vi "Calculator.vi"() -> ()   [LabVIEW 2014]
panel:
  in  ".":bool
  in  "=":bool
  in  "0":bool
  in  "3":bool
  in  "2":bool
  in  "1":bool
  in  "6":bool
  in  "+":bool
  in  "5":bool
  in  "4":bool
  in  "9":bool
  in  "-":bool
  in  "8":bool
  in  "7":bool
  in  "/":bool
  in  "*":bool
  in  "+/-":bool
  in  "C":bool
  in  "M-":bool
  in  "MR":bool
  in  "M+":bool
  in  "MC":bool
  out "?":dbl
  # "Calculator"
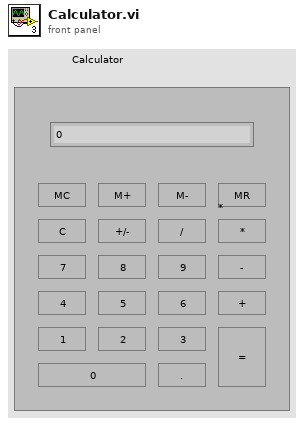
[diagram p1: front panel]
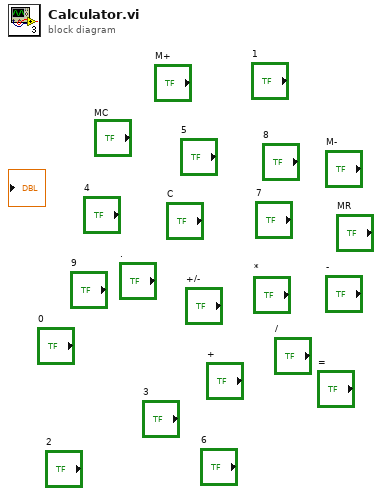
[diagram p0: block diagram]
diagram:
